vi "A33ConfigureTrigger_py.vi"(1 "Trigger Source (0: Immediate)":i32(ring)=2 items=["Immediate (Burst period)", "Timer", "External", "Software Trigger Function"], 2 "Trigger Level (0.9-3.8V)":dbl=2.0 format="%#_12g", 5 "Channel (1: Channel1)":u16(ring)=1 items=["Channel1"=1, "Channel2"=2], 7 "Int period (1 s)":dbl=1.0 format="%#_12g", 9 "Delay (0 s)":dbl format="%#_12g", 12 "Trigger Slope (0: Positive)":u16(ring) items=["Positive", "Negative"]) -> ()   [LabVIEW 2022 SP3]
doc: "Configures the trigger source for triggering sweeps.\n\n<B>Note:</B> Use this VI only with other low-level VIs. The high-level VIs automatically incorporate this functionality. This VI does not check the instrument status. If you want to check the instrument status, call the Error Query VI at the conclusion of your sweep operation."
uses:
  <vilib>/addons/zeromq/zmq_socket.lvclass
panel:
  out "Standalone":bool
  out "socket out":refnum<class "zmq_socket.lvclass">
  in  "socket in":refnum<class "zmq_socket.lvclass">
  out "error out":errorcluster
  out "resulting string":string
  in  "Instrument":string
  in  "error in (no error)":errorcluster
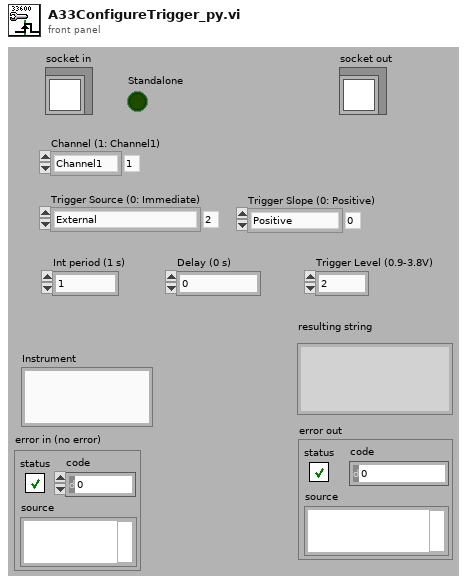
[diagram p1: front panel]
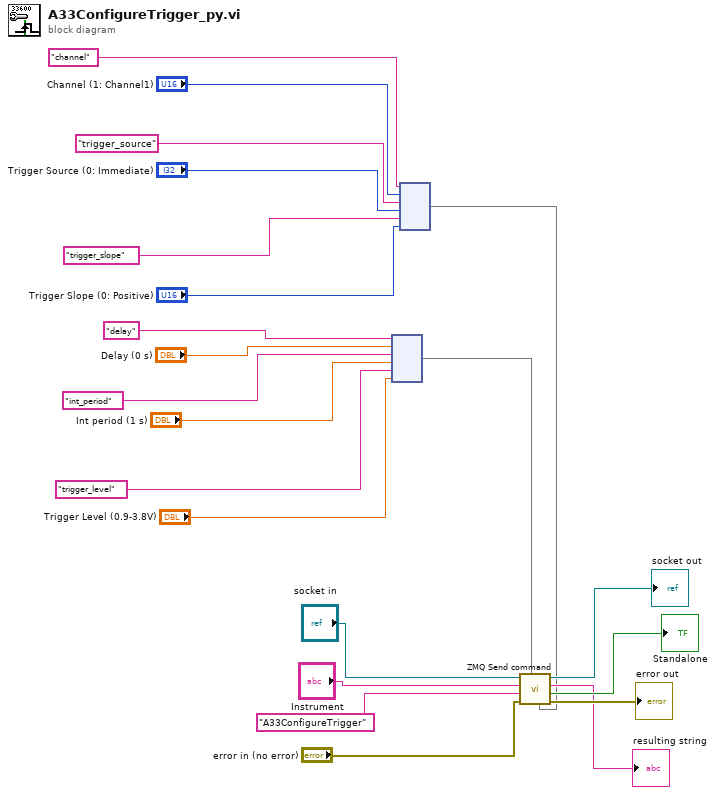
[diagram p0: block diagram]
diagram:
  n1 = node("delay" ("key"), "Delay (0 s)", "int_period" ("key"), "Int period (1 s)", "trigger_level" ("key"), "Trigger Level (0.9-3.8V)") -> (w11:map{string, dbl})
  n2 = node("channel" ("key"), "Channel (1: Channel1)", "trigger_source" ("key"), "Trigger Source (0: Immediate)", "trigger_slope" ("key"), "Trigger Slope (0: Positive)") -> (w10:map{string, i32})
  n3 = call "ZMQ Send command.vi"("Int args"=w10, "DBL args"=w11, "error in"="error in (no error)", "Command"="A33ConfigureTrigger", "Instrument"="Instrument", "socket in"="socket in") -> ("error out"=→"error out":errorcluster, "Standalone"=→"Standalone":bool, "Recieved message"=→"resulting string":string, "socket out"=→"socket out":refnum<class "zmq_socket.lvclass">)  [unwired: 2 in]
